vi "Create Fast Grid.vi"(8 "error in (no error)":errorcluster, 10 "3D Plot.lvclass in":refnum<class "3D Plot.lvclass">, 11 "Fast Draw Object In":refnum<vi>) -> (0 "error out":errorcluster, 2 "3D Plot.lvclass out":refnum<class "3D Plot.lvclass">, 3 "Fast Draw Object Out":refnum<vi>)   [LabVIEW 2020, in "3D Plot.lvclass"]
uses:
  3D Plot.lvclass
  Tick Array.ctl
  3D Plot.lvclass/3D Plot.ctl
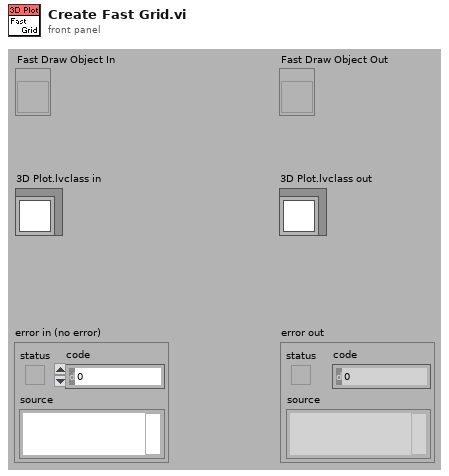
[diagram p1: front panel]
types:
  T1 = typedef "3D Plot.lvclass/Tick Array.ctl" = cluster{"Label":bool, "Show Tick":bool, "Show Line":bool, "Value Numeric":sgl, "Value String":string}[]
  T2 = cluster{"Draw Grid Plane X-Y":bool, "Draw Grid Plane Y-Z":bool, "Draw Grid Plane X-Z":bool}
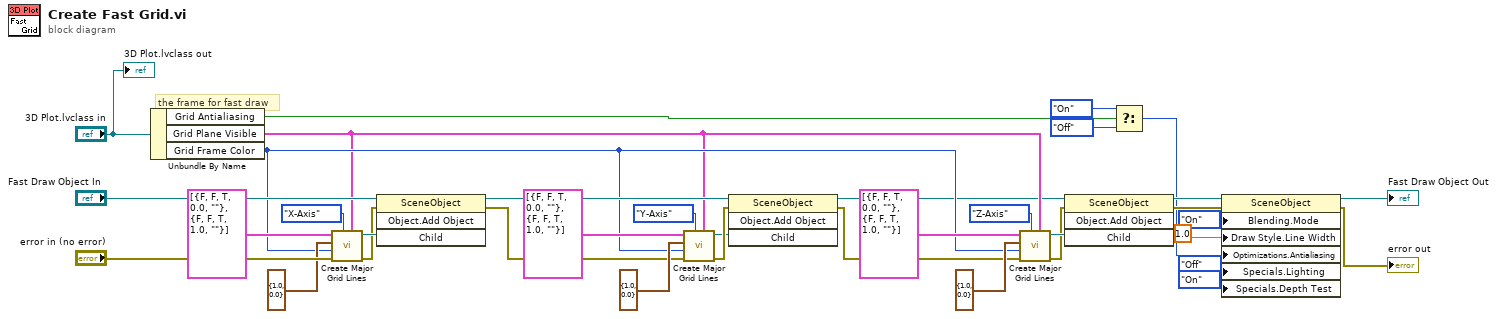
[diagram p0: block diagram]
diagram:
  # "the frame for fast draw"
  n1 = Unbundle By Name("3D Plot.lvclass in") -> ("Grid Antialiasing"=w1:bool, "Grid Plane Visible"=w12:T2, "Grid Frame Color"=w13:u32)
  n2 = call "Create Major Grid Lines.vi"("Grid Plane Visible"=w12, "Axis"=enum16{"X-Axis", "Y-Axis", "Z-Axis"}."X-Axis", "error in (no error)"="error in (no error)", "Grid Color"=w13, "Range"=cluster{sgl, sgl} {1.0, 0.0}, "Tick Cluster Array"=T1 [{"Label"=FALSE, "Show Tick"=FALSE, "Show Line"=TRUE, "Value Numeric"=0.0, "Value String"=""}, {"Label"=FALSE, "Show Tick"=FALSE, "Show Line"=TRUE, "Value Numeric"=1.0, "Value String"=""}]) -> ("error out"=w27:errorcluster, "Grid Object Out"=w28:refnum<vi>)  [unwired: 2 in, 2 out]
  n3 = invoke class="SceneObject" method="Object.Add Object"(reference="Fast Draw Object In", error in=w27, "Child"=w28) -> (reference out=w21:refnum<vi>, error out=w20:errorcluster)  [unwired: 1 in, 2 out]
  n4 = call "Create Major Grid Lines.vi"("Grid Plane Visible"=w12, "Axis"=enum16{"X-Axis", "Y-Axis", "Z-Axis"}."Y-Axis", "error in (no error)"=w20, "Grid Color"=w13, "Range"=cluster{sgl, sgl} {1.0, 0.0}, "Tick Cluster Array"=T1 [{"Label"=FALSE, "Show Tick"=FALSE, "Show Line"=TRUE, "Value Numeric"=0.0, "Value String"=""}, {"Label"=FALSE, "Show Tick"=FALSE, "Show Line"=TRUE, "Value Numeric"=1.0, "Value String"=""}]) -> ("error out"=w26:errorcluster, "Grid Object Out"=w25:refnum<vi>)  [unwired: 2 in, 2 out]
  n5 = invoke class="SceneObject" method="Object.Add Object"(reference=w21, error in=w26, "Child"=w25) -> (reference out=w11:refnum<vi>, error out=w14:errorcluster)  [unwired: 1 in, 2 out]
  n6 = call "Create Major Grid Lines.vi"("Grid Plane Visible"=w12, "Axis"=enum16{"X-Axis", "Y-Axis", "Z-Axis"}."Z-Axis", "error in (no error)"=w14, "Grid Color"=w13, "Range"=cluster{sgl, sgl} {1.0, 0.0}, "Tick Cluster Array"=T1 [{"Label"=FALSE, "Show Tick"=FALSE, "Show Line"=TRUE, "Value Numeric"=0.0, "Value String"=""}, {"Label"=FALSE, "Show Tick"=FALSE, "Show Line"=TRUE, "Value Numeric"=1.0, "Value String"=""}]) -> ("error out"=w15:errorcluster, "Grid Object Out"=w16:refnum<vi>)  [unwired: 2 in, 2 out]
  n7 = invoke class="SceneObject" method="Object.Add Object"(reference=w11, error in=w15, "Child"=w16) -> (reference out=w6:refnum<vi>, error out=w5:errorcluster)  [unwired: 1 in, 2 out]
  n8 = Select(t=enum16{"Inherit Value", "Off", "On"}."On" ("Optimizations:Antialiasing"), s=w1, f=enum16{"Inherit Value", "Off", "On"}."Off" ("Optimizations:Antialiasing")) -> (s? t:f=w2:enum16{"Inherit Value", "Off", "On"})
  n9 = property class="SceneObject"(reference=w6, error in=w5, "Blending.Mode"=enum16{"Inherit Value", "Off", "On"}."On" ("Specials:Lighting"), "Draw Style.Line Width"=sgl 1.0 ("Draw Style:Line Width"), "Optimizations.Antialiasing"=w2, "Specials.Lighting"=enum16{"Inherit Value", "Off", "On"}."Off" ("Blending:Mode"), "Specials.Depth Test"=enum16{"Inherit Value", "Off", "On"}."On" ("Specials:Depth Test")) -> (reference out=→"Fast Draw Object Out":refnum<vi>, error out=→"error out":errorcluster)
  "3D Plot.lvclass out" <- "3D Plot.lvclass in"
